vi "Determine VI Type.vi"(8 "error in":errorcluster, 11 "SubVI Ref in":refnum<vi>) -> (0 "error out":errorcluster, 2 "Instance VI Type":T1, 3 "SubVI Ref out":refnum<vi>)   [LabVIEW 2020, in "Peek Window.lvlib" / "Standard VI Type.lvclass"]
uses:
  Standard VI Type.lvclass
  VI Types Enum.ctl
  Standard VI Type.lvclass/Standard VI Type.ctl
  Malleable VI Type/Malleable VI Type.lvclass
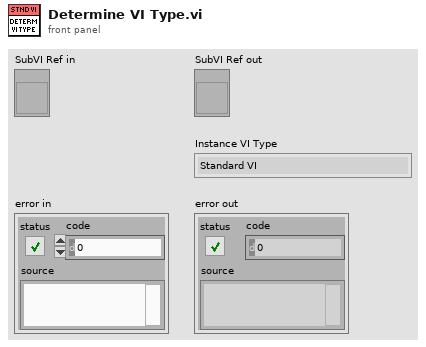
[diagram p1: front panel]
types:
  T1 = typedef "Peek Window.lvlib/Standard VI Type.lvclass/VI Types Enum.ctl" = enum16{"Standard VI", "Malleable VI", "Express VI", "Dynamic Dispatch VI", "Polymorphic VI", "Missing VI"}
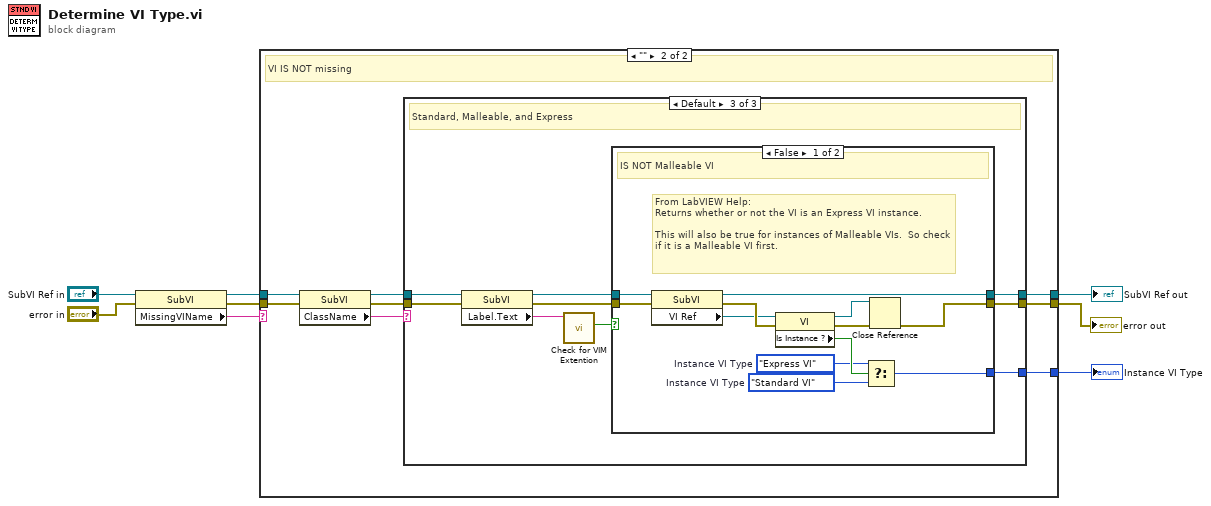
[diagram p0: block diagram]
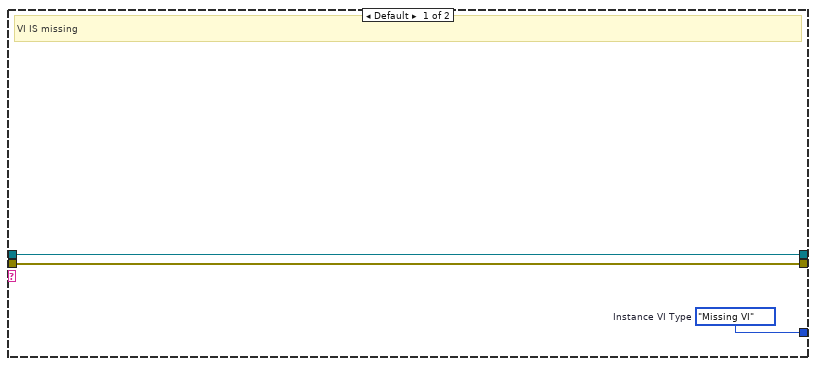
[diagram p2: hidden frame]
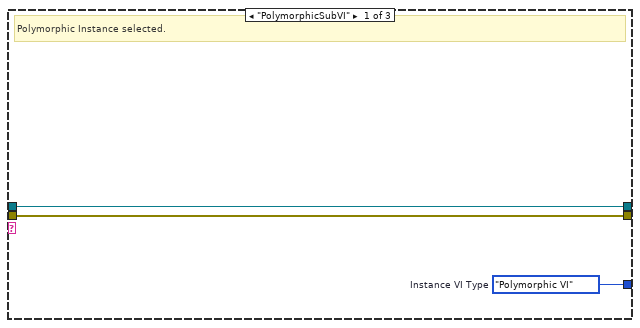
[diagram p3: hidden frame]
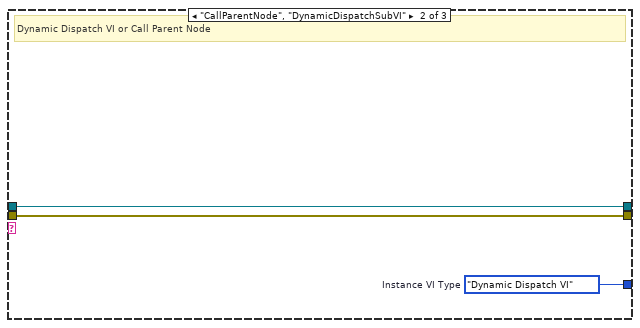
[diagram p4: hidden frame]
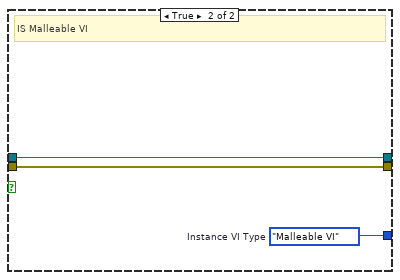
[diagram p5: hidden frame]
diagram:
  n1 = property class="SubVI"(reference="SubVI Ref in", error in="error in") -> (reference out=w2:refnum<vi>, error out=w4:errorcluster, "MissingVIName"=w1:string)
  n2 = case shown="\"\"" w1 {
    tunnel: [w10 w19] -> w7
    tunnel: [w11 w18] -> w6
    tunnel: [w9 w17] -> w5
    tunnel: w4 -> [w10 w15]
    tunnel: w2 -> [w11 w16]
    frame Default {
      w9 = VI_Types_Enum."Missing VI"  # Instance VI Type
      # "VI IS missing"
    }
    frame "" {
      # "VI IS NOT missing"
      n3 = property class="SubVI"(reference=w16, error in=w15) -> (reference out=w14:refnum<vi>, error out=w13:errorcluster, "ClassName"=w12:string)
      n4 = case shown="Default" w12 {
        tunnel: [w21 w24 w32] -> w19
        tunnel: [w22 w25 w29] -> w18
        tunnel: [w20 w23 w28] -> w17
        tunnel: w14 -> [w22 w25 w27]
        tunnel: w13 -> [w21 w24 w26]
        frame "PolymorphicSubVI" {
          w20 = VI_Types_Enum."Polymorphic VI"  # Instance VI Type
          # "Polymorphic Instance selected."
        }
        frame "CallParentNode", "DynamicDispatchSubVI" {
          w23 = VI_Types_Enum."Dynamic Dispatch VI"  # Instance VI Type
          # "Dynamic Dispatch VI or Call Parent Node"
        }
        frame Default {
          # "Standard, Malleable, and Express"
          n5 = property class="SubVI"(reference=w27, error in=w26) -> (reference out=w30:refnum<vi>, error out=w33:errorcluster, "Label.Text"=w34:string)
          n6 = call "Check for VIM Extention.vi"("VI Name in"=w34) -> ("Is a Malleable VI"=w31:bool)  [unwired: 9 in, 1 out]
          n7 = case shown="False" w31 {
            tunnel: w33 -> [w44 w47]
            tunnel: [w43 w47] -> w32
            tunnel: w30 -> [w37 w48]
            tunnel: [w36 w48] -> w29
            tunnel: [w38 w46] -> w28
            frame False {
              w39 = VI_Types_Enum."Standard VI"  # Instance VI Type
              w40 = VI_Types_Enum."Express VI"  # Instance VI Type
              # "From LabVIEW Help:\nReturns whether or not the VI is an Express VI instance.\n\nThis will also be true for instances of Malleable VIs.  So check if it is a Malleable VI first."
              # "IS NOT Malleable VI"
              n8 = property class="SubVI"(reference=w37) -> (reference out=w36:refnum<vi>, "VI Ref"=w35:refnum<vi>)  [unwired: 1 in, 1 out]
              n9 = property class="VI"(reference=w35, error in=w44) -> (reference out=w42:refnum<vi>, error out=w45:errorcluster, "Is Instance ?"=w41:bool)
              n10 = Select(t=w40, s=w41, f=w39) -> (s? t:f=w38:T1)
              n11 = Close Reference(reference=w42, error in (no error)=w45) -> (error out=w43:errorcluster)
            }
            frame True {
              w46 = VI_Types_Enum."Malleable VI"  # Instance VI Type
              # "IS Malleable VI"
            }
          }
        }
      }
    }
  }
  "error out" <- w7
  "SubVI Ref out" <- w6
  "Instance VI Type" <- w5
